vi "GetAttribute1.vi"(0 "reference in":refnum<class "G#SubClass2.lvclass">, 5 "error in (no error)":errorcluster) -> (12 "Locked":bool, 14 "reference out":refnum<class "G#SubClass2.lvclass">, 15 "Base class.Numeric":dbl, 16 "SubAttribute":dbl, 17 "Base class.Array":dbl[](array[numeric]), 19 "error out":errorcluster)   [LabVIEW 2020, in "G#SubClass2.lvclass"]
uses:
  G#SubClass2.lvclass
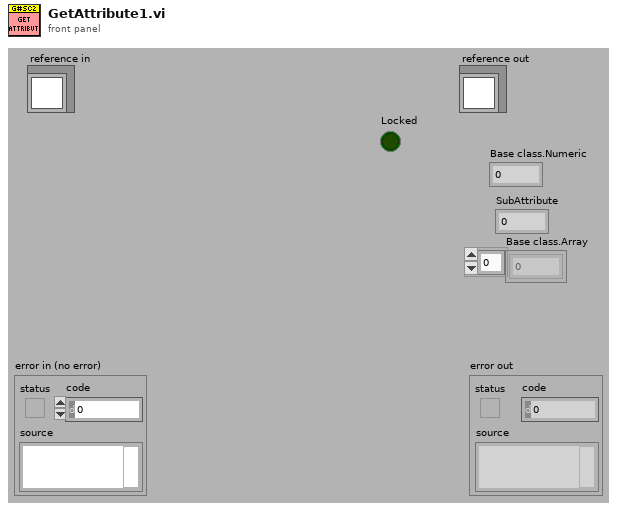
[diagram p1: front panel]
types:
  T1 = typedef "G#SubClass2.lvclass/ObjectAttributes.ctl" = cluster{"Base class":T2, "SubAttribute":dbl}
  T2 = typedef "G#BaseClass2.lvclass/ObjectAttributes.ctl" = cluster{"Numeric":dbl, "Array":dbl[]}
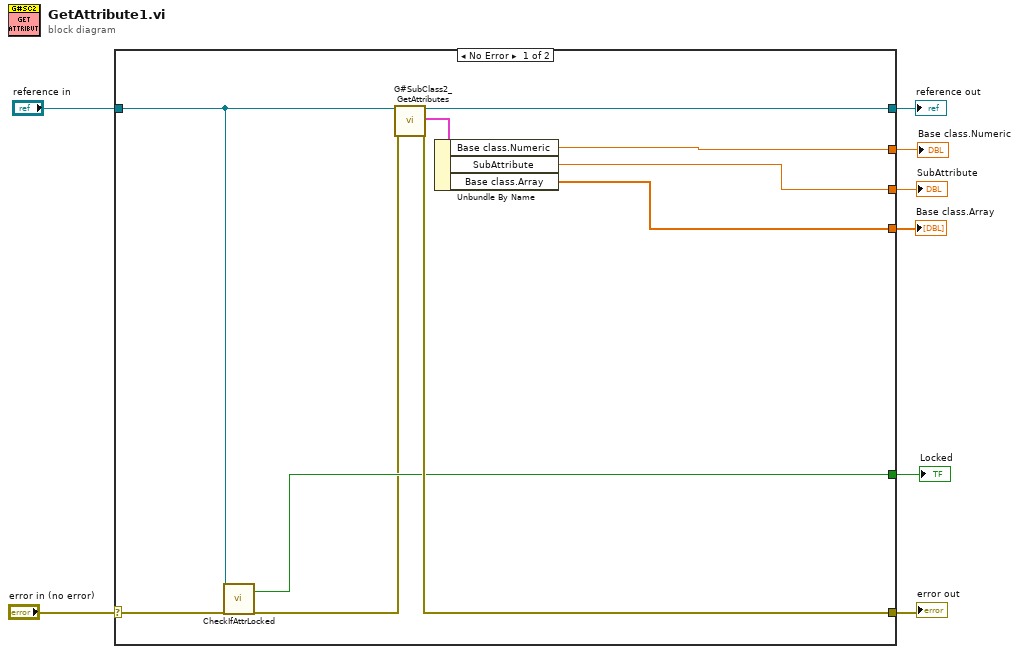
[diagram p0: block diagram]
diagram:
  n1 = case shown="No Error" "error in (no error)" {
    selector: "error in (no error)" -> [w12 w20]
    tunnel: [w17 w20] -> w7
    tunnel: [w16 w19] -> w5
    tunnel: "reference in" -> [w11 w19]
    tunnel: [w10 _] -> w4
    tunnel: [w15 _] -> w3
    tunnel: [w14 _] -> w2
    tunnel: [w13 _] -> w1
    frame No Error {
      n2 = call-dynamic "CheckIfAttrLocked.vi"("reference in"=w11, "error in (no error)"=w12) -> ("locked"=w10:bool, "error out"=w9:errorcluster)  [unwired: 15 in, 1 out]
      n3 = call "G#SubClass2_GetAttributes.vi"("reference in"=w11, "error in (no error)"=w9) -> ("reference out"=w16:refnum<class "G#SubClass2.lvclass">, "attributes"=w18:T1, "error out"=w17:errorcluster)  [unwired: 14 in, 1 out]
      n4 = Unbundle By Name(w18) -> ("Base class.Numeric"=w15:dbl, "SubAttribute"=w14:dbl, "Base class.Array"=w13:dbl[])
    }
    frame Error {
    }
  }
  "error out" <- w7
  "reference out" <- w5
  "Base class.Numeric" <- w3
  "SubAttribute" <- w2
  "Base class.Array" <- w1
  "Locked" <- w4
